vi "Test Flatten Unflatten.vi"() -> ()   [LabVIEW 2019, in "Instrument.Lockin.lvlib" / "Instrument.DAQ.lvclass"]
uses:
  Instrument.DAQ.lvclass
  Instrument.Lockin/Typedefs/API/Lockin.Commands.Local--Enum.ctl
  2c981935-a583-4ceb-b5c1-ecc972d7cc14.vi
  cdec5d56-4ba6-42fd-a6cf-973e75188a99.vi
  <vilib>/JDP Science/JSONtext/Make JSON Array.vi
  cdec5d56-4ba6-42fd-a6cf-973e75188a99.vi/d4123485-b76c-4477-8a19-355dfb4ebc74.vi
  <vilib>/JDP Science/JSONtext/Variant to JSON Text.vi
  <vilib>/JDP Science/JSONtext/support/Format JSON Array Text.vi
  <vilib>/JDP Science/JSONtext/JSON text to Variant.vi
  <vilib>/JDP Science/JSONtext/LVClass Serializer/JSONtext LVClass Serializer.lvclass
  Instrument.Lockin/Instrument.Lockin.lvclass
panel:
  out "error out 2":errorcluster={"status"=TRUE, "code"=116, "source"="Unflatten From String in Test Flatten Unflatten.vi"}
  out "Data out":T1(array[cluster])
  out "data 2":T1(array[cluster])
  out "error out":errorcluster={"status"=TRUE, "code"=116, "source"="Unflatten From String in Test Flatten Unflatten.vi"}
  out "x = y?":bool=TRUE
  out "data":string
  out "variant":variant
  out "data string":string
  in  "DAQ.Config []":T1(array[cluster])=[{"Device"="", "AO.Ch"="", "AO.Range"=enum."±0.1", "AI.Ch"="", "AI.Range"=enum."±0.316", "AI.Coupling"=10050}, {"Device"="", "AO.Ch"="", "AO.Range"=enum."±0.1", "AI.Ch"="", "AI.Range"=enum."±0.316", "AI.Coupling"=10045}] {"AI.Coupling" items=["AC"=10045, "DC"=10050, "GND"=10066]}
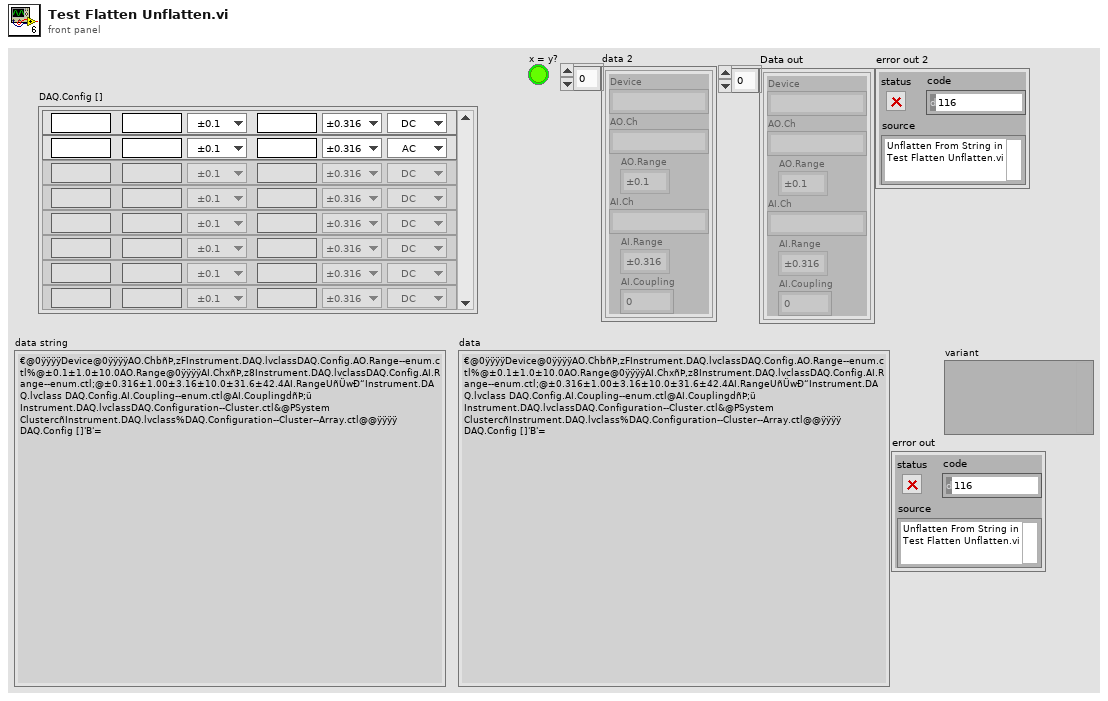
[diagram p1: front panel]
types:
  T1 = cluster{"Device":string, "AO.Ch":string, "AO.Range":enum16{"±0.1", "±1.0", "±10.0"}, "AI.Ch":string, "AI.Range":enum16{"±0.316", "±1.00", "±3.16", "±10.0", "±31.6", "±42.4"}, "AI.Coupling":u16}[]
  T2 = enum16{"big-endian, network order", "native, host order", "little-endian"}
  T3 = typedef "Instrument.Lockin.lvlib/Instrument.Lockin.lvclass/Lockin.Commands.Local--Enum.ctl" = enum16{"autoConfigureDAQ", "setSimulationMode", "setAUX", "zeroPhase", "setCalibration", "setPreFilter", "setLinkFrequencies", "setLimitAmplitude", "setSamplingDecimationPreDSP", "setSamplingDecimationPostDSP", "setSamplingMode", "setSamplingFsMultiplier", "setSamplingFsOutput", "setSamplingRefreshRate", "setData_State", "setData_DAQ", "setData_Sampling", "setData_Waveforms", "setData_Results", "setData_SweepWaveforms", "setData_AIChannels", "setData_AOChannels", "setData_REFChannels", "setData_InputGain", "setData_OutputGain", "showUI", "setAI", "setOffset"}
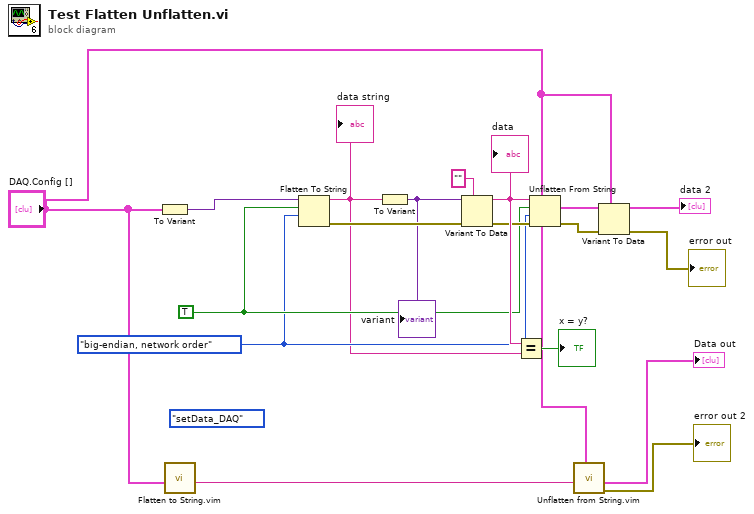
[diagram p0: block diagram]
diagram:
  w8 = TRUE ("prepend array or string size? (T)")
  w7 = T2."big-endian, network order" ("byte order (0:big-endian, network order)")
  (unwired) Lockin.Commands.Local--Enum."setData_DAQ" ("Enum")
  n1 = To Variant(anything="DAQ.Config []") -> (Variant=w9:variant)
  n2 = call "Flatten to String.vim"("Data in"="DAQ.Config []") -> ("<JSON>"=w2:string)  [unwired: 9 in, 1 out]
  n3 = Flatten To String(anything=w9, prepend array or string size? (T)=w8, byte order (0:big-endian, network order)=w7) -> (data string=w1:string, error out=w12:errorcluster)  [unwired: 1 in, 1 out]
  "data string" <- w1
  n4 = To Variant(anything=w1) -> (Variant=w6:variant)
  "variant" <- w6
  n5 = Variant To Data(error in=w12, type="", Variant=w6) -> (data=w15:string, error out=w13:errorcluster)
  "data" <- w15
  n6 = Equal?(x=w15, y=w1) -> (x = y?=→"x = y?":bool)
  n7 = Unflatten From String(type="DAQ.Config []", binary string=w15, data includes array or string size? (T)=w8, byte order (0:big-endian, network order)=w7, error in (no error)=w13) -> (value=w17:T1, error out=w11:errorcluster)  [unwired: 1 out]
  n8 = call "Unflatten from String.vim"("type"="DAQ.Config []", "<JSON>"=w2) -> ("error out"=→"error out 2":errorcluster, "Data out"=→"Data out":T1)  [unwired: 8 in]
  n9 = Variant To Data(error in=w11, type="DAQ.Config []", Variant=w17) -> (data=→"data 2":T1, error out=→"error out":errorcluster)
